vi "enable_motor.vi"(8 "error in (no error)":errorcluster caption="错误输入（无错误）", 11 "StepMotor输入":refnum<class "StepMotor.lvclass">) -> (0 "error out":errorcluster caption="错误输出", 3 "StepMotor输出":refnum<class "StepMotor.lvclass">)   [LabVIEW 2016, in "MotionControl_UFO_3DOF.lvlib" / "StepMotor.lvclass"]
uses:
  <userlib>/MotionControl_UFO_3DOF/StepMotor/StepMotor.lvclass
  <userlib>/MotionControl_UFO_3DOF/StepMotor/StepMotor.lvclass/StepMotor.ctl
  <userlib>/UISimCanFunc_wrapper/UISimCanFunc_wrapper.lvlib
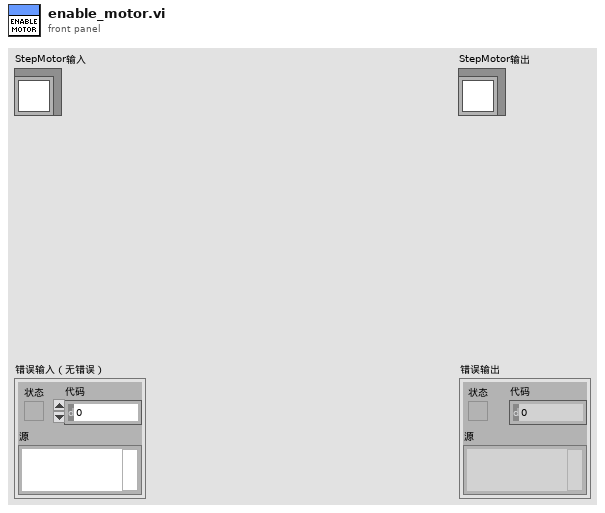
[diagram p1: front panel]
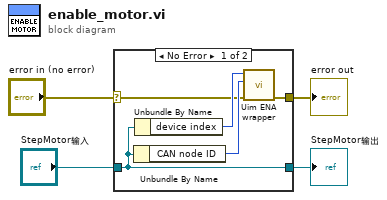
[diagram p0: block diagram]
diagram:
  n1 = case shown="No Error" "error in (no error)" {
    selector: "error in (no error)" -> [w7 w10]
    tunnel: [w6 w10] -> w3
    tunnel: [w5 w11] -> w1
    tunnel: "StepMotor输入" -> [w5 w11]
    frame No Error {
      n2 = Unbundle By Name(w5) -> ("CAN node ID"=w8:u32)
      n3 = Unbundle By Name(w5) -> ("device index"=w9:u32)
      n4 = call <userlib>:"Uim ENA wrapper.vi"("error in (no error)"=w7, "dwCanNodeId"=w8, "dwDevIndex"=w9) -> ("error out"=w6:errorcluster)  [unwired: 6 in, 2 out]
    }
    frame Error {
    }
  }
  "error out" <- w3
  "StepMotor输出" <- w1
